vi "Popup with timeout.vi"(8 "error":errorcluster, 10 "timeout":u32, 11 "message":string) -> (0 "error out":errorcluster)   [LabVIEW 2013]
panel:
  in  "Boolean":bool
  out "String":string
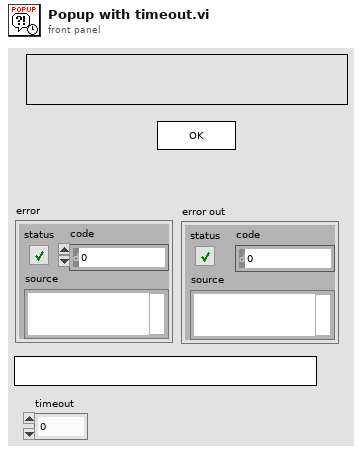
[diagram p1: front panel]
types:
  T1 = enum32{"Invalid", "Standard", "Closed", "Hidden", "Minimized", "Maximized"}
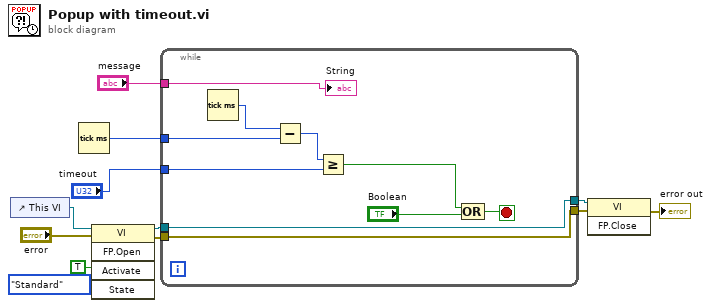
[diagram p0: block diagram]
diagram:
  n1 = control-ref of="This VI"() -> (w7:refnum<vi>)
  n2 = Tick Count (ms)() -> (millisecond timer value=w12:u32)
  n3 = invoke class="VI" method="FP.Open"(reference=w7, error in="error", "Activate"=TRUE ("Activate?"), "State"=T1."Standard") -> (reference out=w4:refnum<vi>, error out=w6:errorcluster)  [unwired: 1 in, 3 out]
  n4 = while {
    tunnel: w12 -> [w21]
    tunnel: "timeout" -> [w19]
    tunnel: [w15] -> w10
    tunnel: w6 -> [w15]
    tunnel: [w14] -> w5
    tunnel: w4 -> [w14]
    tunnel: "message" -> [w13]
    stop <- w16 stop-if-true
    n5 = Tick Count (ms)() -> (millisecond timer value=w22:u32)
    n6 = Subtract(x=w22, y=w21) -> (x-y=w20:u32)
    n7 = Greater Or Equal?(x=w20, y=w19) -> (x >= y?=w18:bool)
    n8 = Compound Arithmetic op=OR(w18, "Boolean") -> (w16:bool)
    "String" <- w13
  }
  n9 = invoke class="VI" method="FP.Close"(reference=w5, error in=w10) -> (error out=→"error out":errorcluster)  [unwired: 1 in, 2 out]
